vi "myRIO v1.0 Open Callback VI.vi"(8 "error in (no error)":errorcluster, 9 "Static Ref in":T1, 11 "Opened VI Ref in":T1) -> (0 "error out":errorcluster, 3 "Opened VI Ref out":T1)   [LabVIEW 2021]
uses:
  <vilib>/myRIO/Common/Instrument Driver Framework/myRIO v1.0/IRQ/typedefs/Callback VI Ref.ctl
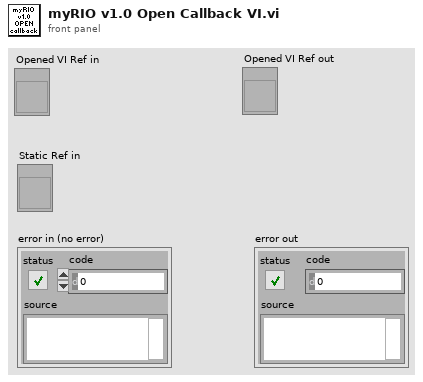
[diagram p1: front panel]
types:
  T1 = typedef "Callback VI Ref.ctl" = refnum<vi>
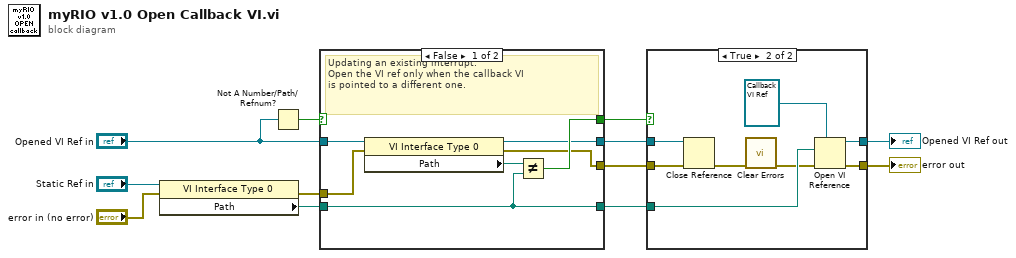
[diagram p0: block diagram]
diagram:
  n1 = property class="VI Interface Type 0"(reference="Static Ref in", error in="error in (no error)") -> (error out=w2:errorcluster, "Path"=w10:path)  [unwired: 1 out]
  n2 = Not A Number/Path/Refnum?(number/path/refnum="Opened VI Ref in") -> (NaN/Path/Refnum?=w12:bool)
  n3 = case shown="False" w12 {
    selector: w12 -> [_ w22]
    tunnel: "Opened VI Ref in" -> [w19 w21]
    tunnel: w2 -> [w14 w23]
    tunnel: [w15 w23] -> w4
    tunnel: [w17 w22] -> w9
    tunnel: w10 -> [w13 w20]
    tunnel: [w16 w21] -> w5
    tunnel: [w13 w20] -> w1
    frame False {
      # "Updating an existing interrupt.\nOpen the VI ref only when the callback VI\nis pointed to a different one."
      n4 = property class="VI Interface Type 0"(reference=w19, error in=w14) -> (reference out=w16:T1, error out=w15:errorcluster, "Path"=w18:path)
      n5 = Not Equal?(x=w18, y=w13) -> (x != y?=w17:bool)
    }
    frame True {
      # "Register a new interrupt.\nIt is OK to open the VI directly."
    }
  }
  n6 = case shown="True" w9 {
    tunnel: w1 -> [_ w32]
    tunnel: [w25 w31] -> w7
    tunnel: [w24 w30] -> w6
    tunnel: w5 -> [w25 w26]
    tunnel: w4 -> [w24 w28]
    frame False {
    }
    frame True {
      n7 = Close Reference(reference=w26, error in (no error)=w28) -> (error out=w29:errorcluster)
      n8 = call <vilib>:"Clear Errors.vi"("error in (no error)"=w29) -> ("error out"=w27:errorcluster)  [unwired: 5 in, 1 out]
      n9 = Open VI Reference(type specifier VI Refnum (for type only)=T1 refnum ("Callback VI Ref"), vi path=w32, error in (no error)=w27) -> (vi reference=w31:T1, error out=w30:errorcluster)  [unwired: 3 in]
    }
  }
  "error out" <- w6
  "Opened VI Ref out" <- w7
